vi "to_linker_info_array.vi"(8 "error in":errorcluster, 11 "HierarchyGraph in":refnum<class "HierarchyGraph.lvclass">) -> (0 "error out":errorcluster, 2 "Linker Info":T1(array[cluster]))   [LabVIEW 2020]
uses:
  HierarchyGraph.lvclass
  api/Graph/Graph.lvclass
  VINode/HierarchyNode.lvclass
  C:/Projects/labview-project-load-tools/source/submodules/graph-api-labview/source/api/Node/Node.lvclass
  C:/Projects/labview-project-load-tools/source/submodules/graph-api-labview/source/example/VINode/HierarchyNode.lvclass
  C:/Projects/labview-project-load-tools/source/submodules/graph-api-labview/source/api/DiGraph/DiGraph.lvclass
  C:/Projects/labview-project-load-tools/source/submodules/graph-api-labview/source/api/Graph/Graph.lvclass
  C:/Projects/labview-project-load-tools/source/submodules/graph-api-labview/source/example/VIGraph/HierarchyGraph.lvclass
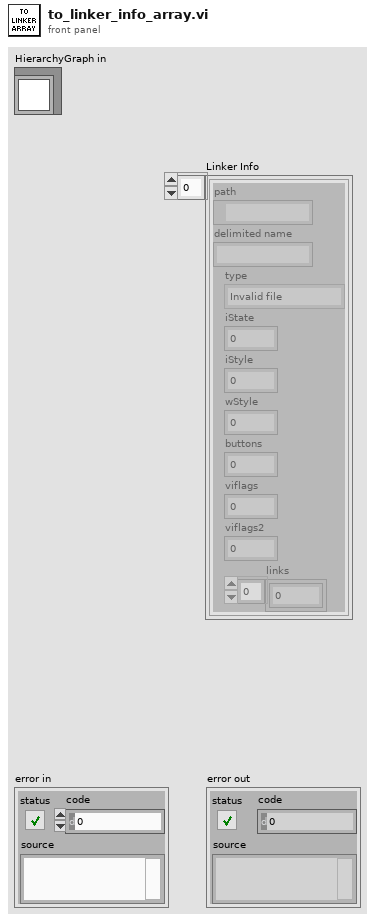
[diagram p1: front panel]
types:
  T1 = cluster{"path":path, "delimited name":string, "type":enum32{"Invalid file", "Unknown type", "Instrument", "Control", "Polymorphic VI", "Project", "Library", "LVClass", "XControl", "XNode", "Shared library", ".NET assembly", "ActiveX interface", "CIN", "Run-time menu", "Palette menu", "Help file", "LLB", "XNode Edit Dependency", "Class Private Data Control", "Statechart", "MathScript .m file", "Ladder Diagram"}, "iState":u32, "iStyle":u16, "wStyle":u16, "buttons":u16, "viflags":u32, "viflags2":u32, "links":u32[]}[]
  T2 = cluster{"path":path, "delimited name":string, "type":enum32{"Invalid file", "Unknown type", "Instrument", "Control", "Polymorphic VI", "Project", "Library", "LVClass", "XControl", "XNode", "Shared library", ".NET assembly", "ActiveX interface", "CIN", "Run-time menu", "Palette menu", "Help file", "LLB", "XNode Edit Dependency", "Class Private Data Control", "Statechart", "MathScript .m file", "Ladder Diagram"}, "iState":u32, "iStyle":u16, "wStyle":u16, "buttons":u16, "viflags":u32, "viflags2":u32, "links":u32[]}
  T3 = enum32{"Invalid file", "Unknown type", "Instrument", "Control", "Polymorphic VI", "Project", "Library", "LVClass", "XControl", "XNode", "Shared library", ".NET assembly", "ActiveX interface", "CIN", "Run-time menu", "Palette menu", "Help file", "LLB", "XNode Edit Dependency", "Class Private Data Control", "Statechart", "MathScript .m file", "Ladder Diagram"}
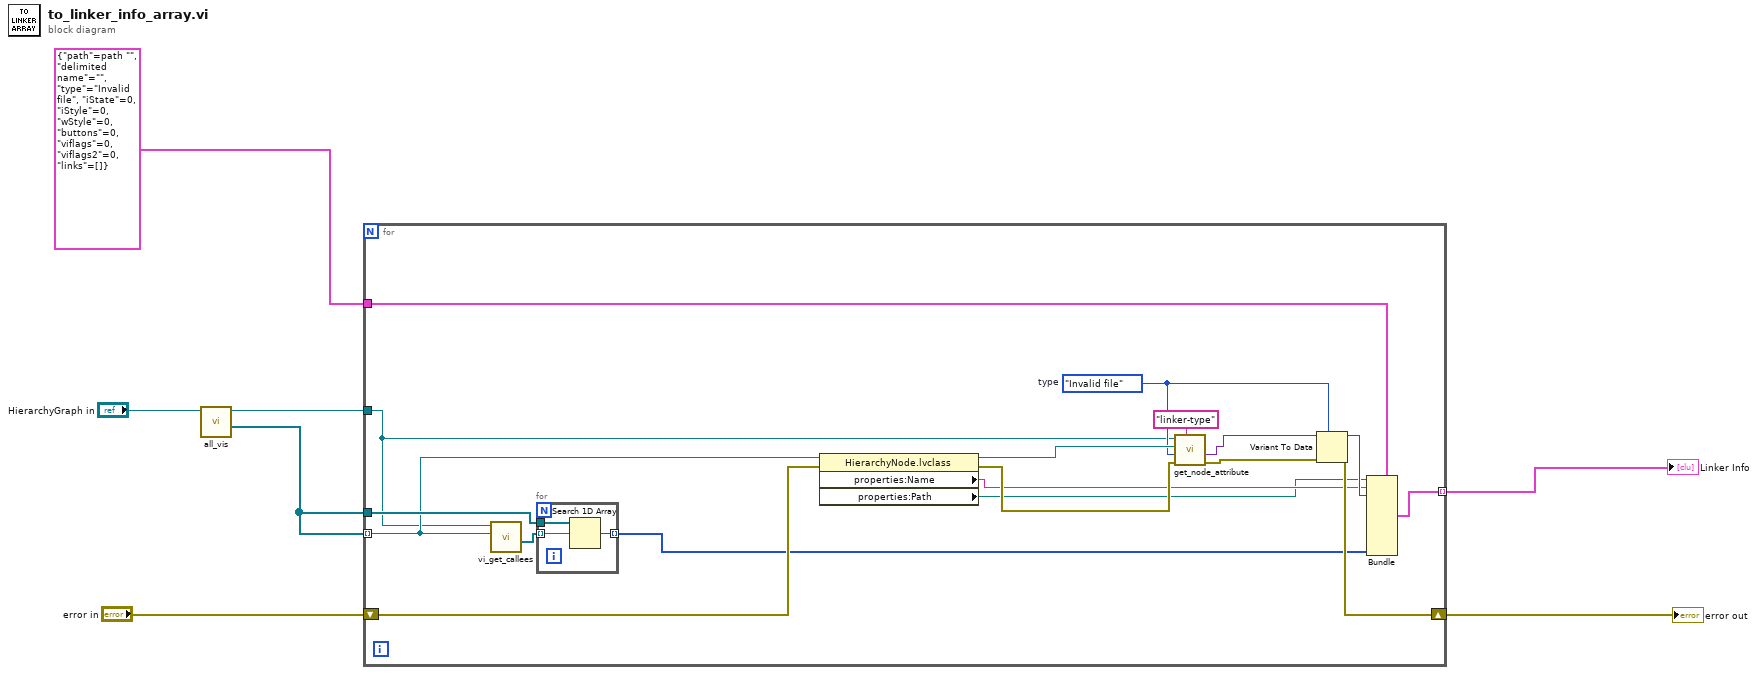
[diagram p0: block diagram]
diagram:
  n1 = call "all_vis.vi"("HierarchyGraph in"="HierarchyGraph in") -> ("VIs"=w2:refnum<class "HierarchyNode.lvclass">[], "HierarchyGraph out"=w3:refnum<class "HierarchyGraph.lvclass">)  [unwired: 8 in, 1 out]
  n2 = for {
    shift-right: [w11] -> w1
    shift-left: "error in" -> [w14]
    tunnel: w2 -> [w19]
    tunnel: w3 -> [w15]
    tunnel: w2 -> [w16] mode=indexing
    tunnel: [w18] -> w5 mode=indexing
    tunnel: T2 {"path"=path "", "delimited name"="", "type"=enum."Invalid file", "iState"=0, "iStyle"=0, "wStyle"=0, "buttons"=0, "viflags"=0, "viflags2"=0, "links"=[]} -> [w17]
    w23 = T3."Invalid file"  # type
    n3 = call "vi_get_callees.vi"("VI"=w16, "Hierarchy"=w15) -> ("Callees"=w21:refnum<class "HierarchyNode.lvclass">[])  [unwired: 8 in, 1 out]
    n4 = for {
      tunnel: w21 -> [w28] mode=indexing
      tunnel: w19 -> [w27]
      tunnel: [w26] -> w10 mode=indexing
      n5 = Search 1D Array(1D array=w27, element=w28) -> (index of element=w26:i32)  [unwired: 1 in]
    }
    n6 = property class="HierarchyNode.lvclass"(reference=w16, error in=w14) -> (reference out=w25:refnum<class "HierarchyNode.lvclass">, error out=w13:errorcluster, "properties:Name"=w9:string, "properties:Path"=w8:path)
    n7 = call "get_node_attribute.vi"("attribute-name"="linker-type", "error in (no error)"=w13, "default value (empty variant)"=w23, "node"=w25, "graph"=w15) -> ("error out"=w12:errorcluster, "attribute-value"=w24:variant)  [unwired: 3 in, 2 out]
    n8 = Variant To Data(error in=w12, type=w23, Variant=w24) -> (data=w22:T3, error out=w11:errorcluster)
    n9 = Bundle(cluster=w17, "path"=w8, "delimited name"=w9, "type"=w22, "links"=w10) -> (w18:T2)  [unwired: 6 in]
  }
  "error out" <- w1
  "Linker Info" <- w5
